vi "状态标记位读写.vi"(5 "更新状态？":bool, 7 "Slave ID":T1=enum."氨氮", 11 "状态":bool) -> (3 "运维标记位":T2)   [LabVIEW 2016, in "质控单元V2.lvlib"]
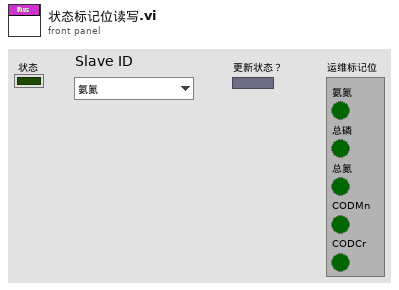
[diagram p1: front panel]
types:
  T1 = typedef "质控单元V2.lvlib/质控slave id.ctl" = enum16{"null", "氨氮", "总磷", "总氮", "CODMn", "CODCr"}
  T2 = cluster{"氨氮":bool, "总磷":bool, "总氮":bool, "CODMn":bool, "CODCr":bool}
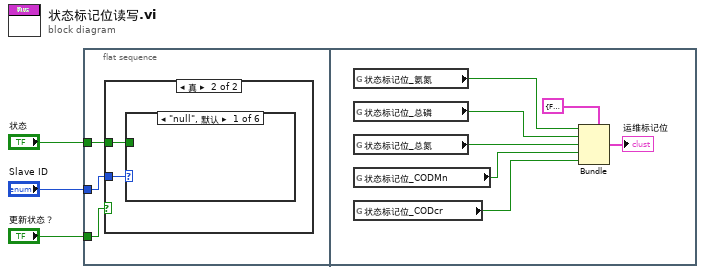
[diagram p0: block diagram]
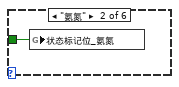
[diagram p3: hidden frame]
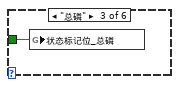
[diagram p4: hidden frame]
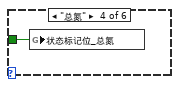
[diagram p5: hidden frame]
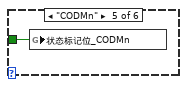
[diagram p6: hidden frame]
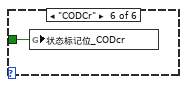
[diagram p7: hidden frame]
diagram:
  n1 = flat-sequence {
    tunnel: "Slave ID" -> [w6]
    tunnel: "状态" -> [w5]
    tunnel: "更新状态？" -> [w4]
    frame #0 {
      n2 = case shown="真" w4 {
        tunnel: w6 -> [_ w8]
        tunnel: w5 -> [_ w7]
        frame False {
        }
        frame True {
          n3 = case shown="\"null\", 默认" w8 {
            tunnel: w7 -> [_ w9 w10 w11 w12 w13]
            frame "null", Default {
            }
            frame "氨氮" {
              n4 = global write "ZK非断电保存全局变量.vi" "状态标记位_氨氮"(w9) -> ()
            }
            frame "总磷" {
              n5 = global write "ZK非断电保存全局变量.vi" "状态标记位_总磷"(w10) -> ()
            }
            frame "总氮" {
              n6 = global write "ZK非断电保存全局变量.vi" "状态标记位_总氮"(w11) -> ()
            }
            frame "CODMn" {
              n7 = global write "ZK非断电保存全局变量.vi" "状态标记位_CODMn"(w12) -> ()
            }
            frame "CODCr" {
              n8 = global write "ZK非断电保存全局变量.vi" "状态标记位_CODcr"(w13) -> ()
            }
          }
        }
      }
    }
    frame #1 {
      n9 = global read "ZK非断电保存全局变量.vi" "状态标记位_氨氮"() -> (w18:bool)
      n10 = global read "ZK非断电保存全局变量.vi" "状态标记位_总磷"() -> (w17:bool)
      n11 = global read "ZK非断电保存全局变量.vi" "状态标记位_总氮"() -> (w16:bool)
      n12 = global read "ZK非断电保存全局变量.vi" "状态标记位_CODMn"() -> (w15:bool)
      n13 = global read "ZK非断电保存全局变量.vi" "状态标记位_CODcr"() -> (w14:bool)
      n14 = Bundle(cluster=T2 {"氨氮"=FALSE, "总磷"=FALSE, "总氮"=FALSE, "CODMn"=FALSE, "CODCr"=FALSE} ("流程运行状态标记位"), "氨氮"=w18, "总磷"=w17, "总氮"=w16, "CODMn"=w15, "CODCr"=w14) -> (→"运维标记位":T2)
    }
  }
